vi "CutDialog.vi"(8 "error in (no error)":errorcluster) -> (0 "error out":errorcluster, 1 "Cancelled":bool, 2 "CommentOut":string, 3 "NameOut":string)   [LabVIEW 2012]
doc: "Asks user for name and comment for new trimmed signal."
panel:
  in  "Cancel Button":bool
  in  "OK Button":bool
  in  "Komentarz":string
  in  "Nazwa sygnału":string
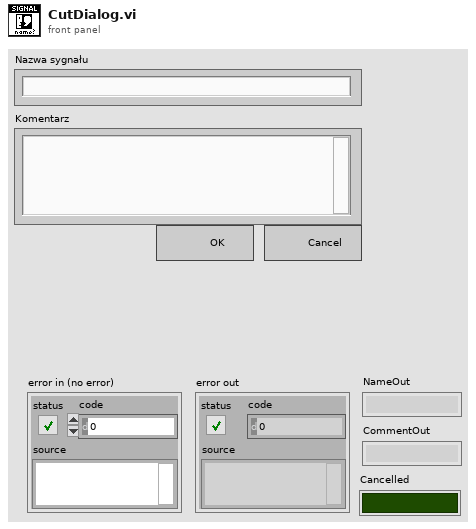
[diagram p1: front panel]
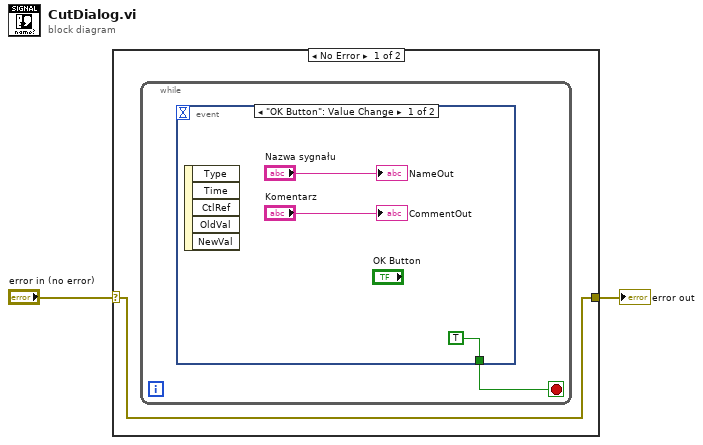
[diagram p0: block diagram]
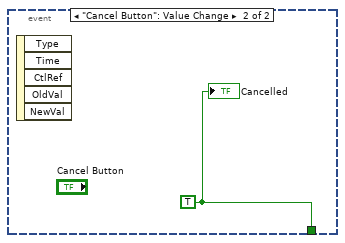
[diagram p2: hidden frame]
diagram:
  n1 = case shown="No Error" "error in (no error)" {
    selector: "error in (no error)" -> [w3 w9]
    tunnel: [w3 w9] -> w1
    frame No Error {
      n2 = while {
        stop <- w4 stop-if-true
        n3 = event shown="[0] \"OK Button\": Value Change" {
          selector: _ -> [_ _]
          dyn-events: _ -> [_ _]
          timeout: _ -> [_ _]
          tunnel: [TRUE w8] -> w4
          event "OK Button": Value Change {
            n4 = event-data() -> ()  [unwired: 1 in, 5 out]
            "NameOut" <- "Nazwa sygnału"
            "CommentOut" <- "Komentarz"
          }
          event "Cancel Button": Value Change {
            w8 = TRUE
            n5 = event-data() -> ()  [unwired: 1 in, 5 out]
            "Cancelled" <- w8
          }
        }
      }
    }
    frame Error {
    }
  }
  "error out" <- w1
